vi "Configure.vi"(8 "error in (no error)":errorcluster, 11 "Test Actors in":refnum<class "Test Actors.lvclass">) -> (0 "error out":errorcluster, 3 "Test Actors out":refnum<class "Test Actors.lvclass">)   [LabVIEW 2015, in "Test Actors.lvclass"]
uses:
  Test Actors.lvclass
  Hardware/LakeShore/Lake Shore Temperature Controller/LakeShore T Controller.lvclass
  Common Measurements/Common Measurements.lvclass
  Mag Lab Measure Base/Mag Lab Measure Base.lvclass
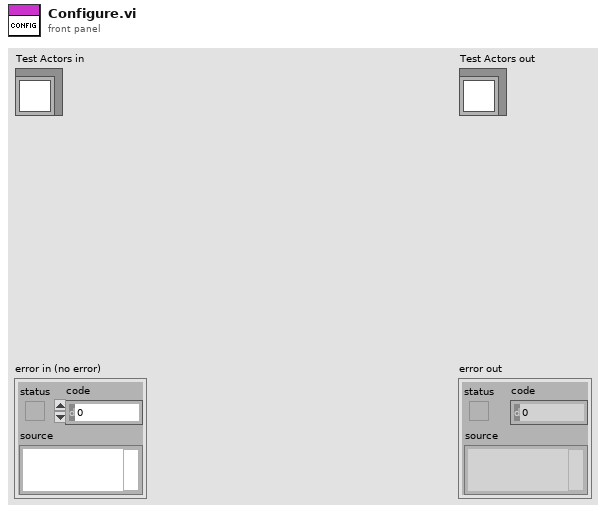
[diagram p1: front panel]
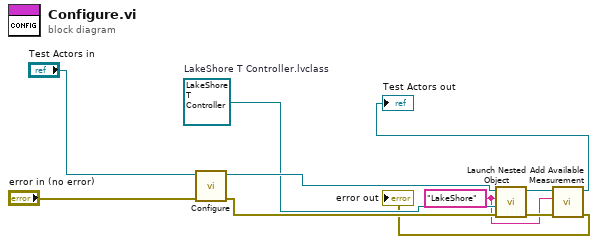
[diagram p0: block diagram]
diagram:
  w3 = "LakeShore" ("name")
  w4 = refnum<class "LakeShore T Controller.lvclass"> refnum  # LakeShore T Controller.lvclass
  n1 = call-parent "Configure.vi"("error in (no error)"="error in (no error)", "Common Measurements in"="Test Actors in") -> ("error out"=w6:errorcluster, "Common Measurements out"=w5:refnum<class "Test Actors.lvclass">)  [unwired: 8 in]
  n2 = call "Launch Nested Object.vi"("error in (no error)"=w6, "Object"=w4, "name"=w3, "Mag Lab Measure Base in"=w5) -> ("error out"=w8:errorcluster, "Mag Lab Measure Base out"=w7:refnum<class "Test Actors.lvclass">)  [unwired: 5 in, 1 out]
  n3 = call-dynamic "Add Available Measurement.vi"("error in (no error)"=w8, "Name"=w3, "Common Measurements in"=w7) -> ("error out"=→"error out":errorcluster, "Common Measurements out"=→"Test Actors out":refnum<class "Test Actors.lvclass">)  [unwired: 7 in]
